vi "Initialize.vi"(8 "error in (no error)":errorcluster, 11 "Lamp Container in":refnum<class "Lamp Container.lvclass">) -> (0 "error out":errorcluster, 3 "Lamp Container out":refnum<class "Lamp Container.lvclass">)   [LabVIEW 2016, in "Lamp Container.lvclass"]
uses:
  Lamp Container.lvclass
  LED/LED.lvclass
  Quartz/Quartz.lvclass
  Dummy Lamp/Dummy Lamp.lvclass
  Lamp Container.lvclass/Lamp Container.ctl
  ThAr/ThAr.lvclass
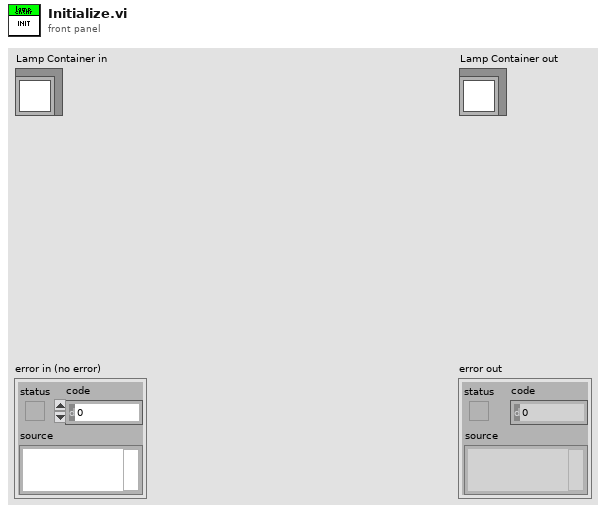
[diagram p1: front panel]
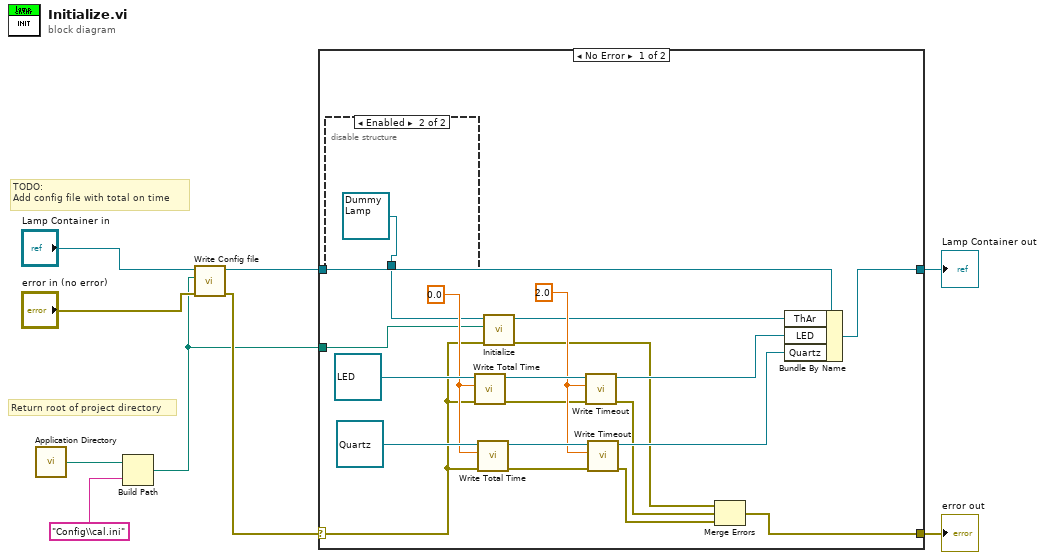
[diagram p0: block diagram]
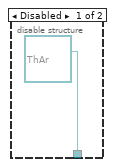
[diagram p2: hidden frame]
diagram:
  # "Return root of project directory"
  # "TODO:\nAdd config file with total on time"
  n1 = call <vilib>:"Application Directory.vi"() -> ("Application Directory"=w3:path)
  n2 = Build Path(base path=w3, name or relative path="Config\\cal.ini") -> (appended path=w1:path)
  n3 = call-dynamic "Write Config file.vi"("error in (no error)"="error in (no error)", "Config file"=w1, "Lamp Container in"="Lamp Container in") -> ("error out"=w4:errorcluster, "Lamp Container out"=w6:refnum<class "Lamp Container.lvclass">)  [unwired: 7 in]
  n4 = case shown="No Error" w4 {
    selector: w4 -> [w15 w33]
    tunnel: [w24 w33] -> w9
    tunnel: [w28 w32] -> w8
    tunnel: w6 -> [w29 w32]
    tunnel: w1 -> [w11 _]
    frame No Error {
      w19 = 2.0 ("Timeout")
      w25 = 0.0
      n5 = disable-structure shown="Enabled" {
        disable-tunnel: [refnum<class "ThAr.lvclass"> refnum ("ThAr.lvclass") refnum<class "Dummy Lamp.lvclass"> refnum ("Dummy Lamp.lvclass")] -> w10
        frame Disabled {
        }
        frame Enabled {
        }
      }
      n6 = call-dynamic "Write Total Time.vi"("error in (no error)"=w15, "Total Time"=w25, "Lamp in"=refnum<class "LED.lvclass"> refnum ("LED.lvclass")) -> ("error out"=w17:errorcluster, "Lamp out"=w23:refnum<class "LED.lvclass">)  [unwired: 7 in]
      n7 = call-dynamic "Write Total Time.vi"("error in (no error)"=w15, "Total Time"=w25, "Lamp in"=refnum<class "Quartz.lvclass"> refnum ("Quartz.lvclass")) -> ("error out"=w18:errorcluster, "Lamp out"=w21:refnum<class "Quartz.lvclass">)  [unwired: 7 in]
      n8 = call-dynamic "Initialize.vi"("error in (no error)"=w15, "config path"=w11, "Lamp in"=w10) -> ("error out"=w12:errorcluster, "Lamp out"=w14:refnum<class "Dummy Lamp.lvclass">)  [unwired: 7 in]
      n9 = call-dynamic "Write Timeout.vi"("error in (no error)"=w17, "Timeout"=w19, "Lamp in"=w23) -> ("error out"=w13:errorcluster, "Lamp out"=w22:refnum<class "LED.lvclass">)  [unwired: 7 in]
      n10 = call-dynamic "Write Timeout.vi"("error in (no error)"=w18, "Timeout"=w19, "Lamp in"=w21) -> ("error out"=w16:errorcluster, "Lamp out"=w20:refnum<class "Quartz.lvclass">)  [unwired: 7 in]
      n11 = Merge Errors(w12, w13, w16) -> (w24:errorcluster)
      n12 = Bundle By Name(cluster=w29, "ThAr"=w14, "LED"=w22, "Quartz"=w20) -> (w28:refnum<class "Lamp Container.lvclass">)
    }
    frame Error {
    }
  }
  "error out" <- w9
  "Lamp Container out" <- w8
